vi "Ventilation_Automation_Project.vi"() -> ()   [LabVIEW 2021]
uses:
  <vilib>/Instr/_visa.llb/VISA Configure Serial Port (Instr).vi
  <vilib>/smtpClient/Set Message Text.vi
  <vilib>/smtpClient/LabVIEWSMTPClient.lvlib
panel:
  out "Bilgilendirme Paneli":string
  out "Gaz miktarı değişimi":dbl(graph)
  out "Eşik değer uyarısı":bool
  out "Okunan değer":dbl
  in  "stop":bool
  in  "Baud Rate":u32=9600
  in  "COM Port":refnum<visa-resource-name>
  # "Havalandırma Kontrol Otomasyonu"
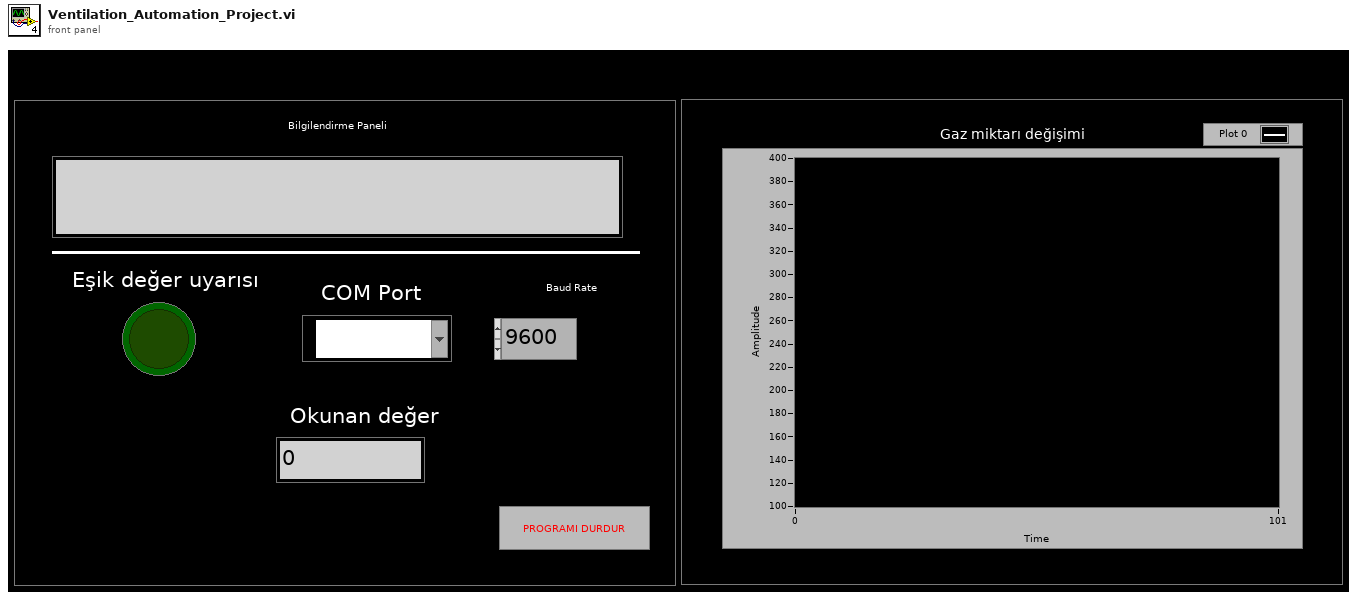
[diagram p1: front panel]
types:
  T1 = typedef "LabVIEWSMTPClient.lvlib/SmtpClientHandle.ctl" = refnum<k1>
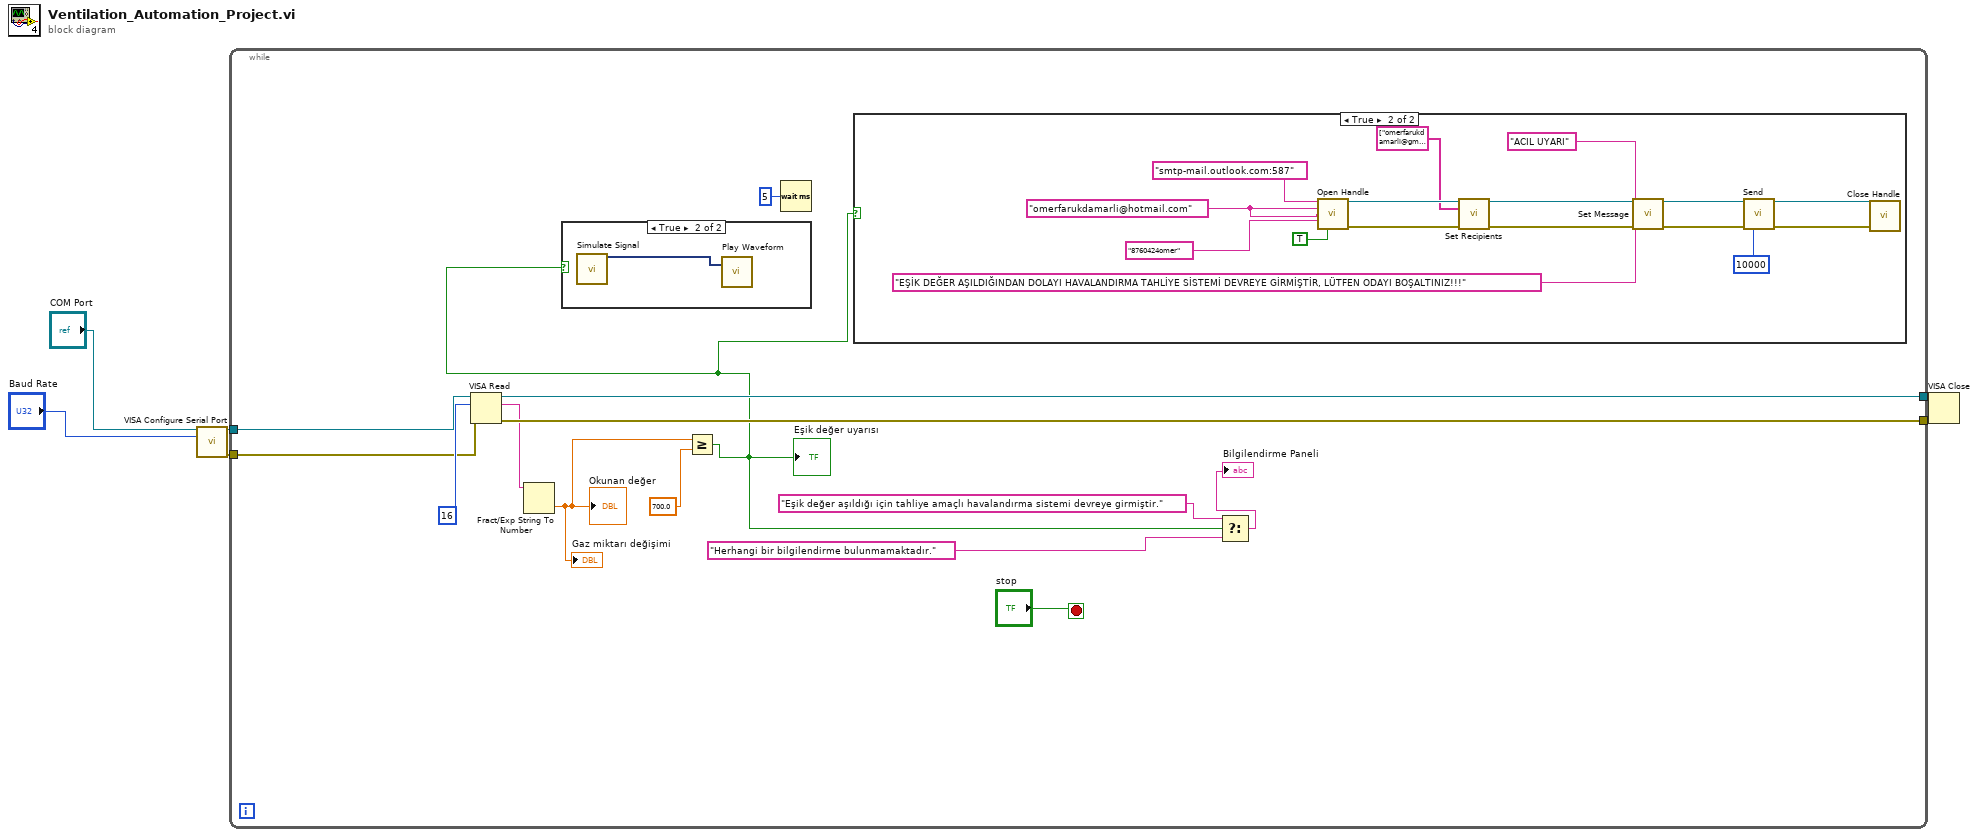
[diagram p0: block diagram]
diagram:
  n1 = call-poly "VISA Configure Serial Port"("VISA resource name"="COM Port", "baud rate (9600)"="Baud Rate") -> ("VISA resource name out"=w4:refnum<visa-resource-name>, "error out"=w2:errorcluster)  [unwired: 12 in]
  n2 = while {
    tunnel: w4 -> [w19]
    tunnel: [w17] -> w3
    tunnel: w2 -> [w16]
    tunnel: [w15] -> w1
    stop <- "stop" stop-if-true
    n3 = VISA Read(VISA resource name=w19, byte count=u32 16, error in (no error)=w16) -> (VISA resource name out=w15:refnum<visa-resource-name>, read buffer=w14:string, error out=w17:errorcluster)  [unwired: 1 out]
    n4 = Fract/Exp String To Number(string=w14) -> (number=w13:dbl)  [unwired: 3 in, 1 out]
    "Okunan değer" <- w13
    "Gaz miktarı değişimi" <- w13
    n5 = Greater Or Equal?(x=w13, y=700.0) -> (x >= y?=w7:bool)
    "Eşik değer uyarısı" <- w7
    n6 = case shown="True" w7 {
      frame False {
      }
      frame True {
        n7 = call "Simulate Signal"() -> ("Sine"=w37:dynamicdata)  [unwired: 14 in, 1 out]
        n8 = call "Play Waveform"("Data"=w37) -> ()  [unwired: 18 in, 1 out]
      }
    }
    n9 = Wait (ms)(milliseconds to wait=u32 5) -> ()  [unwired: 1 out]
    n10 = case shown="True" w7 {
      frame False {
      }
      frame True {
        w27 = "omerfarukdamarli@hotmail.com" ("from")
        n11 = call <vilib>:"Open Handle.vi"("server address"="smtp-mail.outlook.com:587", "from"=w27, "username"=w27, "password"="8760424omer", "use TLS (false)"=TRUE) -> ("handle out"=w36:T1, "error out"=w32:errorcluster)  [unwired: 9 in]
        n12 = call <vilib>:"Set Recipients.vi"("handle in"=w36, "to"=string[] ["omerfarukdamarli@gmail.com"], "error in (no error)"=w32) -> ("handle out"=w35:T1, "error out"=w31:errorcluster)  [unwired: 11 in]
        n13 = call-poly <vilib>:"Set Message.vi"("handle in"=w35, "subject"="ACIL UYARI", "plain text message"="EŞİK DEĞER AŞILDIĞINDAN DOLAYI HAVALANDIRMA TAHLİYE SİSTEMİ DEVREYE GİRMİŞTİR, LÜTFEN ODAYI BOŞALTINIZ!!!", "error in (no error)"=w31) -> ("handle out"=w34:T1, "error out"=w30:errorcluster)  [unwired: 10 in]
        n14 = call <vilib>:"Send.vi"("handle in"=w34, "error in (no error)"=w30, "timeout in ms (10000)"=10000) -> ("handle out"=w33:T1, "error out"=w29:errorcluster)  [unwired: 10 in, 1 out]
        n15 = call <vilib>:"Close Handle.vi"("handle in"=w33, "error in (no error)"=w29) -> ()  [unwired: 12 in, 2 out]
      }
    }
    n16 = Select(t="Eşik değer aşıldığı için tahliye amaçlı havalandırma sistemi devreye girmiştir.", s=w7, f="Herhangi bir bilgilendirme bulunmamaktadır.") -> (s? t:f=→"Bilgilendirme Paneli":string)
  }
  n17 = VISA Close(VISA resource name=w1, error in (no error)=w3) -> ()  [unwired: 1 out]
